vi "Create TCP Connection Handler.vi"(5 "ConnectionHandler in":refnum<class "ConnectionHandler.lvclass">, 8 "error in (no error)":errorcluster, 10 "Connection Configuration":refnum<class "Connection.lvclass">, 11 "Request":refnum<queue>) -> (0 "error out":errorcluster, 3 "ConnectionHandler":refnum<class "ConnectionHandler.lvclass">)   [LabVIEW 2013, in "MQTT_Connection.lvlib" / "ConnectionHandler.lvclass"]
uses:
  ConnectionHandler.lvclass
  MQTT_Base/Base Class/Request -- cluster.ctl
  <vilib>/LabVIEW Open Source Project/MQTT Control Packets/Control Packets/ControlPacket/ControlPacket.lvclass
  MQTT_Base/Base Class/Response -- cluster.ctl
  Connection/Connection.lvclass
  ConnectionHandler.lvclass/ConnectionHandler.ctl
  MQTT_Base/Base Class/MQTT_Base.lvclass
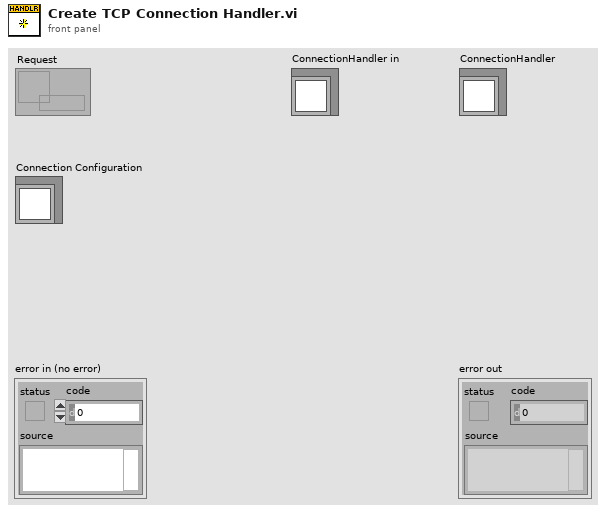
[diagram p1: front panel]
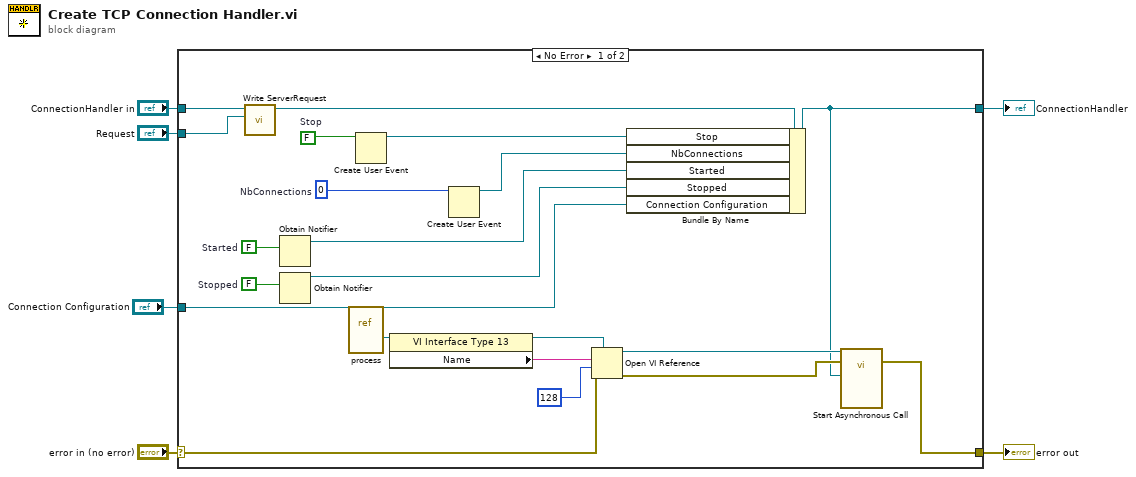
[diagram p0: block diagram]
diagram:
  n1 = case shown="No Error" "error in (no error)" {
    selector: "error in (no error)" -> [w13 w29]
    tunnel: [w12 w29] -> w5
    tunnel: [w16 w28] -> w3
    tunnel: "ConnectionHandler in" -> [w26 w28]
    tunnel: "Request" -> [w27 _]
    tunnel: "Connection Configuration" -> [w7 _]
    frame No Error {
      w11 = u32 0  # NbConnections
      w14 = FALSE  # Stopped
      w15 = FALSE  # Started
      w25 = FALSE  # Stop
      n2 = call "Write ServerRequest.vi"("ServerRequest"=w27, "TCPConnectionHandler in"=w26) -> ("TCPConnectionHandler out"=w23:refnum<class "ConnectionHandler.lvclass">)  [unwired: 9 in]
      n3 = Obtain Notifier(notification data type=w15) -> (notifier out=w9:refnum<notifier>)  [unwired: 3 in, 2 out]
      n4 = Obtain Notifier(notification data type=w14) -> (notifier out=w8:refnum<notifier>)  [unwired: 3 in, 2 out]
      n5 = vi-ref "process.vi"() -> (w22:refnum<vi>)
      n6 = Create User Event(user event datatype=w25) -> (user event=w24:refnum<user-event>)  [unwired: 1 in, 1 out]
      n7 = property class="VI Interface Type 13"(reference=w22) -> (reference out=w20:refnum<vi>, "Name"=w21:string)  [unwired: 1 in, 1 out]
      n8 = Create User Event(user event datatype=w11) -> (user event=w10:refnum<user-event>)  [unwired: 1 in, 1 out]
      n9 = Open VI Reference(type specifier VI Refnum (for type only)=w20, vi path=w21, options=128, error in (no error)=w13) -> (vi reference=w19:refnum<vi>, error out=w18:errorcluster)  [unwired: 2 in]
      n10 = Bundle By Name(cluster=w23, "Stop"=w24, "NbConnections"=w10, "Started"=w9, "Stopped"=w8, "Connection Configuration"=w7) -> (w16:refnum<class "ConnectionHandler.lvclass">)
      n11 = call-by-ref "Start Asynchronous Call"(reference=w19, error in=w18, "ConnectionHandler in"=w16) -> (error out=w12:errorcluster)  [unwired: 9 in, 3 out]
    }
    frame Error {
    }
  }
  "error out" <- w5
  "ConnectionHandler" <- w3
